vi "DC.vi"() -> ()   [LabVIEW 2015]
panel:
  in  "stop":bool
  in  "Power (-100 to 100)\n0 = Stop/Brake\n-128 = Stop/Coast":i8(slide) scale=-100.0..100.0
  in  "Encoder Target: 360 = 1 motor shaft revolution":i32
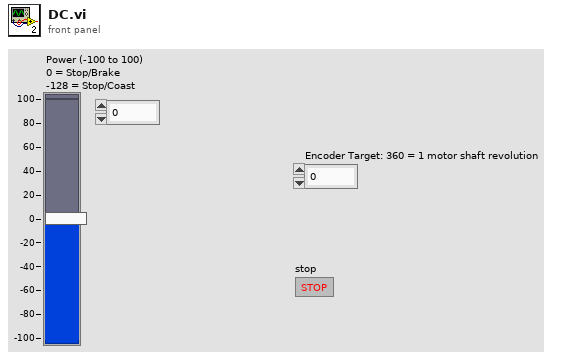
[diagram p1: front panel]
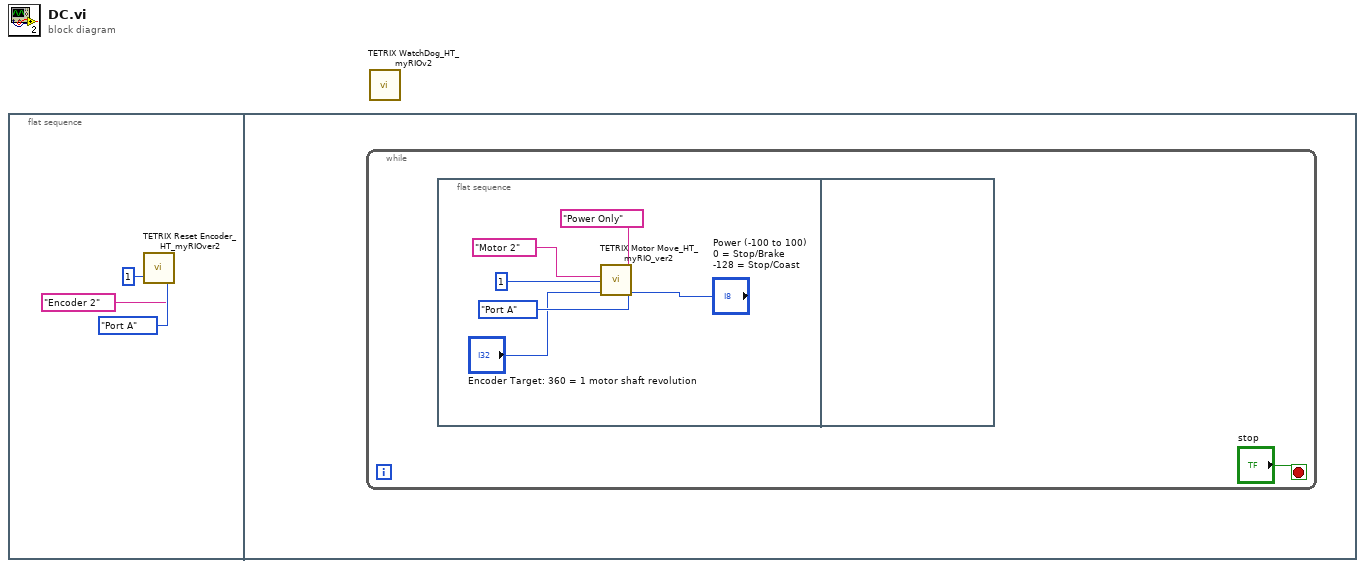
[diagram p0: block diagram]
diagram:
  n1 = flat-sequence {
    frame #0 {
      n2 = call "TETRIX Reset Encoder_HT_myRIOver2.vi"("Controller Daisy Chain Position ( 1 - 4)"=u8 1, "Select Encoder"="Encoder 2", "Port"=enum16{"Port A", "Port B"}."Port A") -> ()  [unwired: 1 in, 1 out]
    }
    frame #1 {
      n3 = while {
        stop <- "stop" stop-if-true
        n4 = flat-sequence {
          frame #0 {
            n5 = call "TETRIX Motor Move_HT_myRIO_ver2.vi"("Select Channel"="Motor 2", "Controller Daisy Chain Position: 1 - 4"=u8 1, "Encoder Target: 360 = 1 motor shaft revolution"="Encoder Target: 360 = 1 motor shaft revolution", "Control Mode"="Power Only", "Port"=enum16{"Port A", "Port B", ""}."Port A", "Power (-100 to 100)\n0 = Stop/Brake\n-128 = Stop/Coast"="Power (-100 to 100)\n0 = Stop/Brake\n-128 = Stop/Coast") -> ()  [unwired: 2 in, 1 out]
          }
          frame #1 {
          }
        }
      }
    }
  }
  n6 = call "TETRIX WatchDog_HT_myRIOv2.vi"() -> ()  [unwired: 4 in]
